vi "Custom Device Input Read.vi"(8 "error in (no error)":errorcluster, 11 "RT data in":T1) -> (0 "error out":errorcluster, 3 "RT data out":T1)   [LabVIEW 2011, in "Engine Sim RT.lvlib"]
uses:
  Engine Sim RT.lvlib
  TypeDefs/RT Data Cluster.ctl
  Shared/Channel Descriptors.ctl
  Shared/FPGA Write Descriptor.ctl
  Shared/InputChannelTypes.ctl
  <vilib>/rvi/DataTransferAndStorage/Container/Common/niFpgaDataTypeControl.ctl
  Shared/FPGA Read Descriptor.ctl
  Shared/OutputChannelTypes.ctl
  Shared/Status Chan Descriptor.ctl
  Shared/DataReplayVoltageConfig.ctl
  Engine Simulation Shared.lvlib
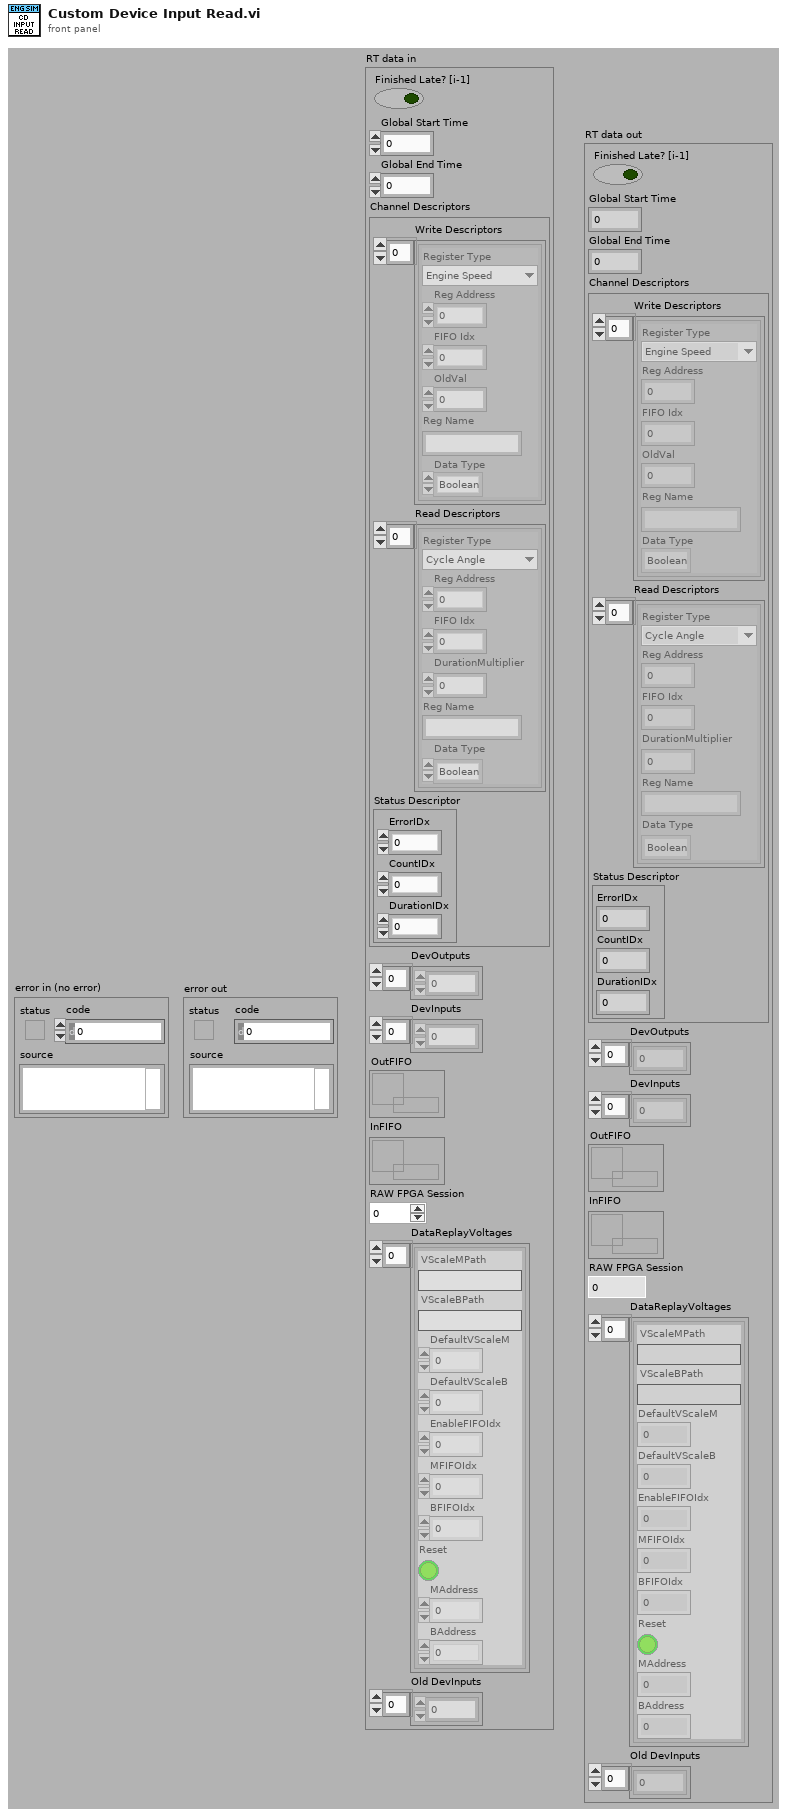
[diagram p1: front panel]
types:
  T1 = typedef "Engine Sim RT.lvlib/RT Data Cluster.ctl" = cluster{"Finished Late? [i-1]":bool, "Global Start Time":i64, "Global End Time":i64, "Channel Descriptors":T2, "DevOutputs":dbl[], "DevInputs":dbl[], "OutFIFO":refnum<k33>, "InFIFO":refnum<k33>, "RAW FPGA Session":u32, "DataReplayVoltages":T9[], "Old DevInputs":dbl[]}
  T2 = typedef "Engine Simulation Shared.lvlib/Channel Descriptors.ctl" = cluster{"Write Descriptors":T3[], "Read Descriptors":T6[], "Status Descriptor":T8}
  T3 = typedef "Engine Simulation Shared.lvlib/FPGA Write Descriptor.ctl" = cluster{"Register Type":T4, "Reg Address":u32, "FIFO Idx":i32, "OldVal":dbl, "Reg Name":string, "Data Type":T5}
  T4 = typedef "Engine Simulation Shared.lvlib/InputChannelTypes.ctl" = enum16{"Engine Speed", "Offset"}
  T5 = typedef "niFpgaDataTypeControl.ctl" = enum32{"Boolean", "I8", "I16", "I32", "I64", "U8", "U16", "U32", "U64", "FXP", "CustomControl"}
  T6 = typedef "Engine Simulation Shared.lvlib/FPGA Read Descriptor.ctl" = cluster{"Register Type":T7, "Reg Address":u32, "FIFO Idx":i32, "DurationMultiplier":dbl, "Reg Name":string, "Data Type":T5}
  T7 = typedef "Engine Simulation Shared.lvlib/OutputChannelTypes.ctl" = enum16{"Cycle Angle", "Crank Angle", "Time Duration", "Angle Duration", "Start Angle", "End Angle"}
  T8 = typedef "Engine Simulation Shared.lvlib/Status Chan Descriptor.ctl" = cluster{"ErrorIDx":i32, "CountIDx":i32, "DurationIDx":i32}
  T9 = typedef "Engine Simulation Shared.lvlib/DataReplayVoltageConfig.ctl" = cluster{"VScaleMPath":string, "VScaleBPath":string, "DefaultVScaleM":u32, "DefaultVScaleB":i32, "EnableFIFOIdx":i32, "MFIFOIdx":i32, "BFIFOIdx":i32, "Reset":bool, "MAddress":u32, "BAddress":u32}
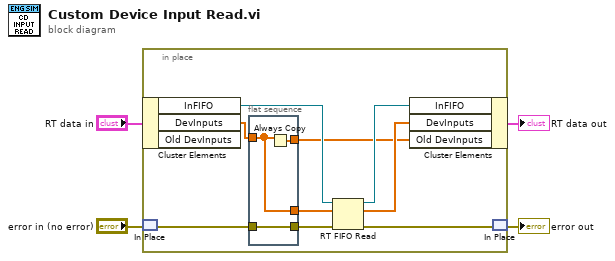
[diagram p0: block diagram]
diagram:
  n1 = in-place {
    n2 = in-place-cluster #1("RT data in") -> ("InFIFO"=w11:refnum<k33>, "DevInputs"=w9:dbl[])  [unwired: 1 out]
    n3 = in-place-match #2("error in (no error)") -> (w6:errorcluster)
    n4 = flat-sequence {
      tunnel: w9 -> [w14]
      tunnel: [w16] -> w8
      tunnel: [w15] -> w7
      tunnel: w6 -> [w15]
      tunnel: [w14] -> w5
      frame #0 {
        n5 = Always Copy(1:w14) -> (0:w16:dbl[])
      }
    }
    n6 = RT FIFO Read(0:w11, 1:w5, 3:w7) -> (8:w10:refnum<k33>, 9:w12:dbl[], 11:w13:errorcluster)  [unwired: 3 out]
    n7 = in-place-cluster #1("InFIFO"=w10, "DevInputs"=w12, "Old DevInputs"=w8) -> (→"RT data out":T1)
    n8 = in-place-match #2(w13) -> (→"error out":errorcluster)
  }
